vi "Detect Barcodes.vi"   [LabVIEW 2020, in "feature_detection.lvlib" / "Barcode Detector.lvclass"]
uses:
  Barcode Detector.lvclass
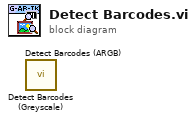
[diagram p0: block diagram]
diagram:
  n1 = call "Detect Barcodes (Greyscale).vi"() -> ()  [unwired: 9 in, 3 out]
  n2 = call "Detect Barcodes (ARGB).vi"() -> ()  [unwired: 9 in, 3 out]
